vi "Z Aux Direct Cambox.vi"(0 "handle":u32, 1 "fDistance":sgl, 2 "ioption":i32, 5 "istartpoint":i32, 7 "iendpoint":i32, 9 "ftablemulti":sgl, 11 "error in (no error)":errorcluster caption="错误输入（无错误）", 12 "ilinkaxis":i32, 13 "flinkstartpos":sgl) -> (4 "handle out":u32, 6 "function return":i32, 15 "error out":errorcluster caption="错误输出")   [LabVIEW 2015, in "zauxdll.lvlib"]
doc: "int32 __stdcall ZAux_Direct_Cambox(ZMC_HANDLE handle, int istartpoint, int iendpoint, float ftablemulti, float fDistance, int ilinkaxis, int ioption, float flinkstartpos);"
uses:
  zauxdll.lvlib
  Radar - 2015 32bit_autoqueue_angle_0319/zauxdll-2014/zauxdll.dll
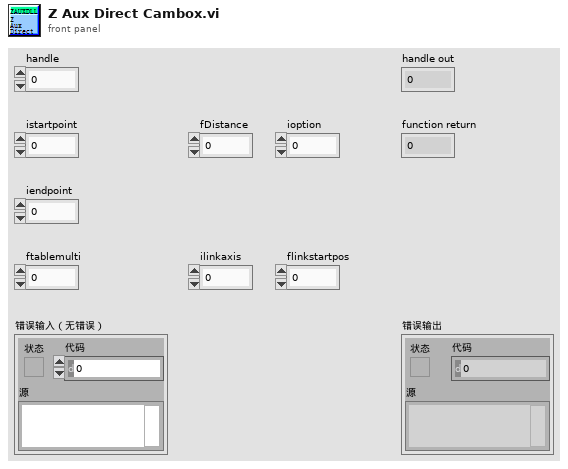
[diagram p1: front panel]
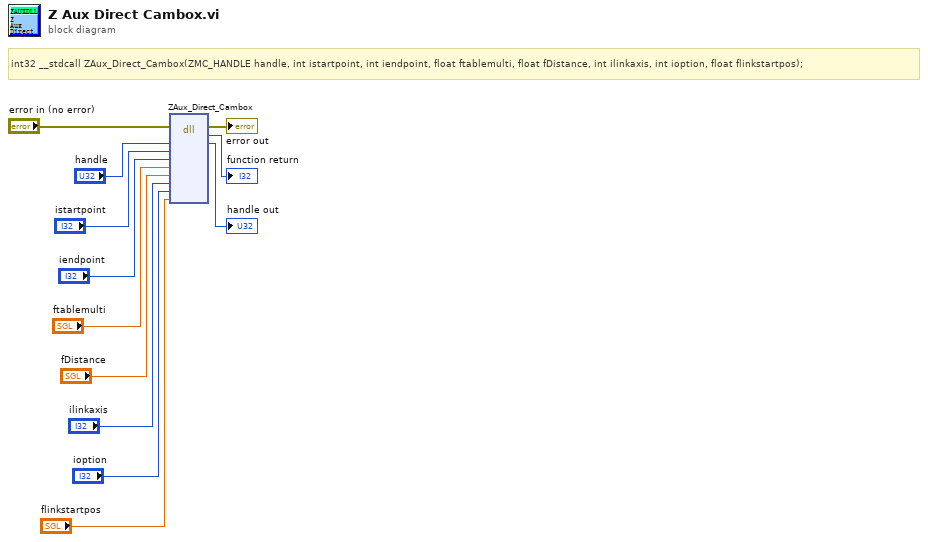
[diagram p0: block diagram]
diagram:
  # "int32 __stdcall ZAux_Direct_Cambox(ZMC_HANDLE handle, int istartpoint, int iendpoint, float ftablemulti, float fDistance, int ilinkaxis, int ioption, float flinkstartpos);"
  n1 = dll-call lib="D:/vicomm case/cub/0717/Radar - 2015 32bit_autoqueue_angle_0319/zauxdll-2014/zauxdll.*" fn="ZAux_Direct_Cambox"(error in="error in (no error)", "handle"="handle", "istartpoint"="istartpoint", "iendpoint"="iendpoint", "ftablemulti"="ftablemulti", "fDistance"="fDistance", "ilinkaxis"="ilinkaxis", "ioption"="ioption", "flinkstartpos"="flinkstartpos") -> (error out=→"error out":errorcluster, →"function return":i32, "handle"=→"handle out":u32)  [unwired: 9 in, 1 out]
